vi "PH_Cam_BaseClass.destructor.vi"(0 "i ref in":refnum<vi>, 5 "error in(no error)":errorcluster) -> (19 "error out":errorcluster)   [LabVIEW 2014, in "PH_Cam_BaseClass.lvlib"]
doc: "This is the destructor of a class.\n\nLicense Agreement for this software:\n\nCopyright (C)\nGesellschaft für Schwerionenforschung, GSI\nPlanckstr. 1\n64291 Darmstadt\nGermany\n\nContact: D.Beck@gsi.de \n\nThis program is free software; you can redistribute it and/or modify it under the terms of the \nGNU General Public License as published by the Free Software Foundation; either version 2 of \nthe license, or (at your option) any later version.\n\nThis program is distributed in the hope that it will be useful, but WITHOUT ANY WARRANTY; \nwithout even the implied warranty of MERCHANTABILITY or FITNESS FOR A PARTICULAR PURPOSE. See the GNU General License for more details (http://www.gnu.org).\n\nGesellschaft für Schwerionenforschung, GSI\nPlanckstr. 1, 64291 Darmstadt, Germany\nFor all questions and ideas contact: M.Richter@gsi.de, H.Brand@gsi.de or D.Beck@gsi.de.\nLast update: 16-JUN-2004"
uses:
  PH_Cam_BaseClass.lvlib
  CSlibraries-extern/DimLVEvent/LVDimInterface/LVDimInterface.lvlib
  PH_PSDBWriter/PH_PSDBWriter.lvlib
  PH_StatusHandler/PH_StatusHandler.lvlib
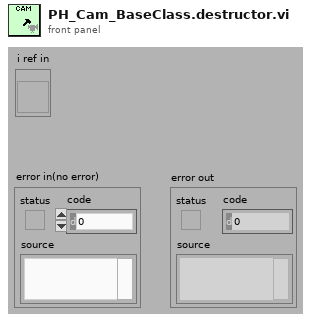
[diagram p1: front panel]
types:
  T1 = typedef "PH_Cam_BaseClass.lvlib/PH_Cam_BaseClass.i attribute.ctl" = cluster{"Gui Refs":T2, "Cam":cluster{"Source Notifier":refnum<notifier>, "Error":errorcluster, "Camera ID":string}, "Images":cluster{"Cam":T3, "Operation":T3, "PSDB":T3}, "Window Image":cluster{"Indicate Image":bool, "Window No.":i32, "Scale Facor":dbl, "Center Cross":bool, "Subtract Backgr":bool, "CoG":bool, "Color Palette":cluster{"Red":u8, "Green":u8, "Blue":u8}[], "Image On":bool}, "Default Prdc Int":i32, "Performance":cluster{"on":bool, "Timestamp Last Frame":i32}, "Histogram":cluster{"on":bool, "Mapping":bool}, "Save Image":cluster{"Save":bool, "File refnum":refnum<file>}, "Setting Service ID":i32, "Screen":cluster{"x-resolution":i16, "y-resolution":i16}, "On":bool, "Constructor finished":bool, "configured":bool}
  T2 = typedef "PH_Cam_BaseClass.lvlib/PH_Cam_BaseClass.GUI Refs.ctl" = cluster{"Frame Rate":refnum<vi>, "Get Frame Rate":refnum<vi>, "Show Image":refnum<vi>, "Get Histogram":refnum<vi>, "Mapping":refnum<vi>, "Histogram":refnum<vi>, "Center Cross":refnum<vi>, "Center of Gravity":refnum<vi>, "Scale Factor [%]":refnum<vi>, "Save Image":refnum<vi>, "Palette":refnum<vi>, "Subtract Background":refnum<vi>, "Cam Error":refnum<vi>, "On":refnum<vi>, "Cam List":refnum<vi>}
  T3 = typedef "IMAQ Image.ctl" = refnum<image>
  T4 = enum16{"SetAttribute", "GetAttribute", "CreateAttribute", "DestroyAttribute", "DestroyAllAtributes"}
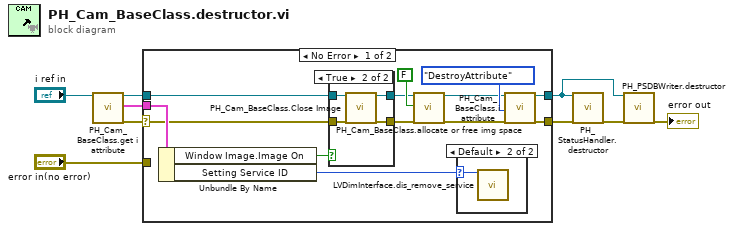
[diagram p0: block diagram]
diagram:
  n1 = call "PH_Cam_BaseClass.get i attribute.vi"("i ref in"="i ref in") -> ("i ref out"=w8:refnum<vi>, "i attribute"=w6:T1, "error out"=w5:errorcluster)  [unwired: 16 in]
  n2 = case shown="No Error" w5 {
    selector: w5 -> [w12 _]
    tunnel: [w19 w30] -> w9
    tunnel: w8 -> [w18 w31]
    tunnel: w6 -> [w17 _]
    tunnel: [w13 w31] -> w1
    tunnel: "error in(no error)" -> [_ w30]
    frame No Error {
      n3 = Unbundle By Name(w17) -> ("Window Image.Image On"=w16:bool, "Setting Service ID"=w21:i32)
      n4 = case shown="True" w16 {
        tunnel: w18 -> [w24 w26]
        tunnel: w12 -> [w23 w25]
        tunnel: [w23 w28] -> w14
        tunnel: [w24 w27] -> w15
        frame False {
        }
        frame True {
          n5 = call "PH_Cam_BaseClass.Close Image.vi"("i ref in"=w26, "error in"=w25) -> ("i ref out"=w27:refnum<vi>, "error out"=w28:errorcluster)  [unwired: 16 in]
        }
      }
      n6 = call "PH_Cam_BaseClass.allocate or free img space.vi"("i ref in"=w15, "Allocate?"=FALSE, "error in (no error)"=w14) -> ("i ref out"=w10:refnum<vi>, "error out"=w11:errorcluster)  [unwired: 15 in]
      n7 = case shown="Default" w21 {
        selector: w21 -> [_ w29]
        frame -1 {
        }
        frame Default {
          n8 = call "LVDimInterface.dis_remove_service.vi"("my_serviceID"=w29) -> ()  [unwired: 18 in, 1 out]
        }
      }
      n9 = call "PH_Cam_BaseClass.i attribute.vi"("VI Refnum"=w10, "Action"=T4."DestroyAttribute", "error in (no error)"=w11) -> ("VI Refnum out"=w13:refnum<vi>, "error out"=w19:errorcluster)  [unwired: 14 in, 1 out]
    }
    frame Error {
    }
  }
  n10 = call "PH_StatusHandler.destructor.vi"("i ref in"=w1, "error in(no error)"=w9) -> ("error out"=w2:errorcluster)  [unwired: 17 in]
  n11 = call "PH_PSDBWriter.destructor.vi"("i ref in"=w1, "error in(no error)"=w2) -> ("error out"=→"error out":errorcluster)  [unwired: 17 in]
